vi "LocalizationFGV.vi"(0 "Action":T1, 1 "Dictionary File Path":path, 5 "VI in":refnum<vi>, 7 "Target Language":string, 9 "Input":string, 11 "error in":errorcluster) -> (4 "CSV String":string, 6 "Dictionary":T2, 8 "Languages":string[](array[string]), 10 "Result":string, 14 "Current Language":string, 15 "error out":errorcluster)   [LabVIEW 2020]
uses:
  Dictionary--Cluster.ctl
  Font -- Cluster.ctl
  Phrase Dictionary Entry -- Cluster.ctl
  Localization FGV Action -- Enum.ctl
  VI Info -- Cluster.ctl
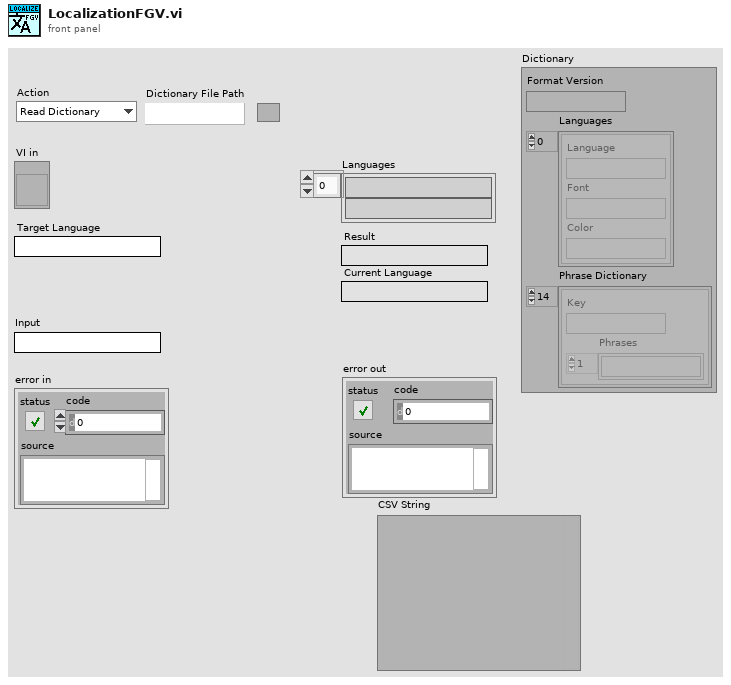
[diagram p1: front panel]
types:
  T1 = typedef "Localization FGV Action -- Enum.ctl" = enum16{"Read Dictionary", "Translate VIs", "Register VI", "Get Languages", "Translate Phrase", "Get Key For Phrase", "Get Phrase For Phrase", "Translate VI", "Unregister"}
  T2 = typedef "Dictionary--Cluster.ctl" = cluster{"Format Version":string, "Languages":T3[], "Phrase Dictionary":T4[]}
  T3 = typedef "Font -- Cluster.ctl" = cluster{"Language":string, "Font":string, "Color":string}
  T4 = typedef "Phrase Dictionary Entry -- Cluster.ctl" = cluster{"Key":string, "Phrases":string[]}
  T5 = typedef "VI Info -- Cluster.ctl" = cluster{"VI Ref":refnum<vi>, "Language":string}
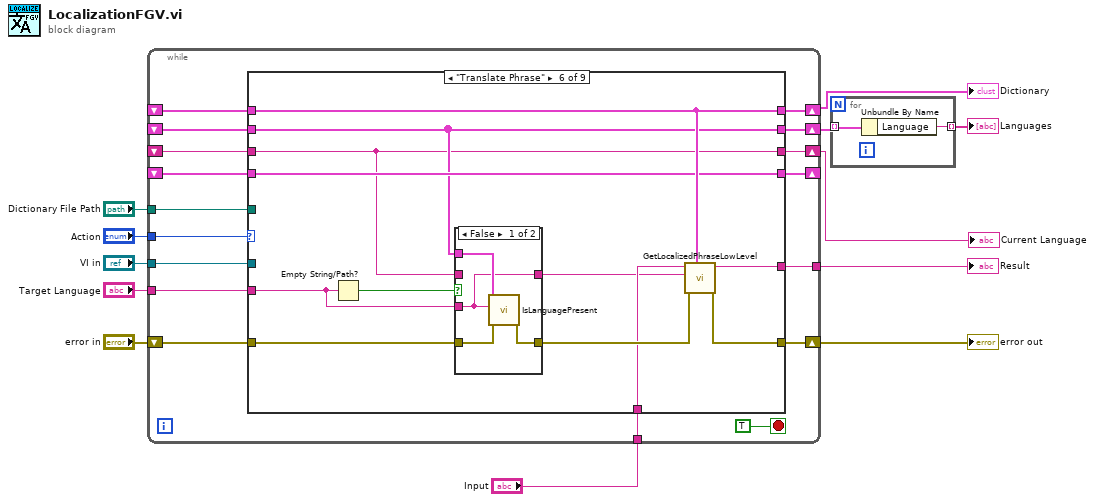
[diagram p0: block diagram]
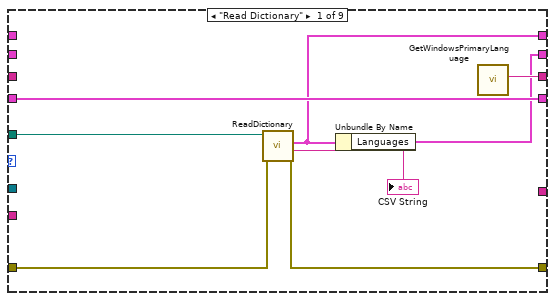
[diagram p2: hidden frame]
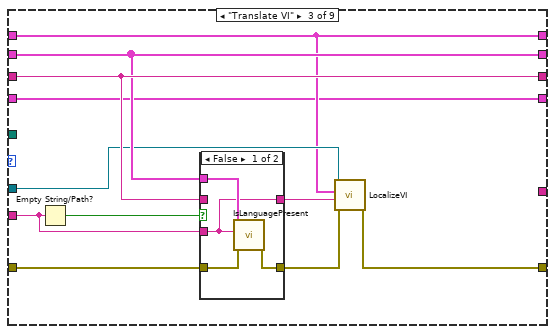
[diagram p4: hidden frame]
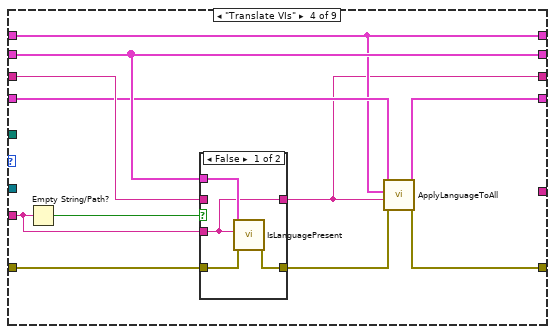
[diagram p6: hidden frame]
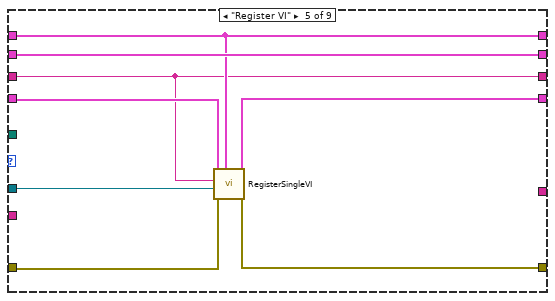
[diagram p8: hidden frame]
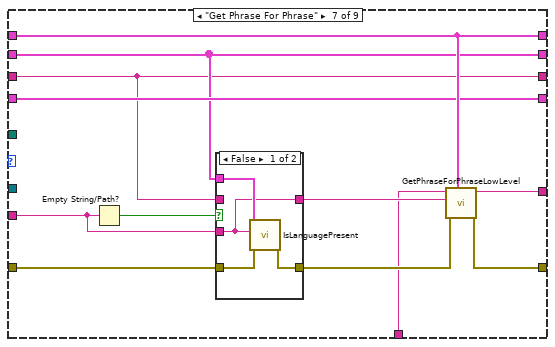
[diagram p10: hidden frame]
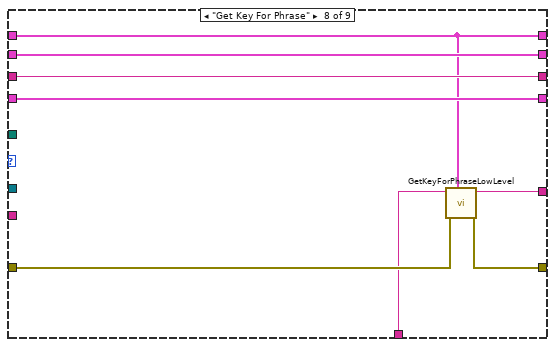
[diagram p12: hidden frame]
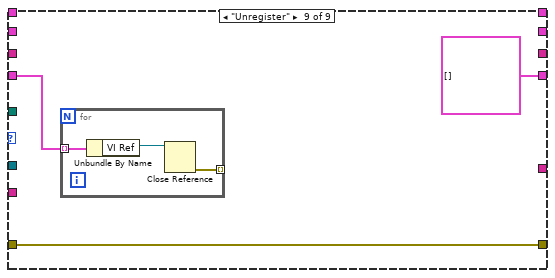
[diagram p13: hidden frame]
diagram:
  n1 = while {
    tunnel: "Action" -> [w28]
    tunnel: "Dictionary File Path" -> [w27]
    shift-right: [w26] -> w4
    shift-left: _ -> [w25]
    shift-right: [w15] -> w11
    shift-left: "error in" -> [w24]
    tunnel: "VI in" -> [w23]
    shift-right: [w22] -> _
    shift-left: _ -> [w21]
    shift-right: [w20] -> w3
    shift-left: _ -> [w19]
    tunnel: "Target Language" -> [w18]
    shift-right: [w17] -> w5
    shift-left: _ -> [w16]
    tunnel: [w14] -> w7
    tunnel: "Input" -> [w13]
    stop <- TRUE stop-if-true
    n2 = case shown="\"Translate Phrase\"" w28 {
      tunnel: w27 -> [w37 _ _ _ _ _ _ _ _]
      tunnel: [w32 w42 w45 w63 w81 w96 w114 w123 _] -> w26
      tunnel: w25 -> [_ w42 w45 w63 w81 w96 w114 w123 _]
      tunnel: w24 -> [w35 w39 w49 w66 w83 w92 w110 w125 w131]
      tunnel: w23 -> [_ _ w46 _ w77 _ _ _ _]
      tunnel: [w34 w40 w43 w64 w79 w94 w112 w128 T5[] [] ("VI Status")] -> w22
      tunnel: w21 -> [w34 w40 w43 w65 w80 w94 w112 w128 w130]
      tunnel: [w31 w41 w50 w67 w84 w90 w108 w127 _] -> w20
      tunnel: w19 -> [_ w41 w50 w67 w84 w90 w108 w127 _]
      tunnel: w18 -> [_ _ w51 w68 _ w89 w106 _ _]
      tunnel: [w33 w38 w52 w60 w78 w88 w105 w126 _] -> w17
      tunnel: w16 -> [_ w38 w52 w69 w78 w88 w105 w126 _]
      tunnel: [w36 w39 w47 w61 w82 w95 w113 w124 w131] -> w15
      tunnel: [_ _ _ _ _ w93 w111 w121 _] -> w14
      tunnel: w13 -> [_ _ _ _ _ w87 w103 w122 _]
      frame "Read Dictionary" {
        n3 = call "ReadDictionary.vi"("error in (no error)"=w35, "Dictionary File Path"=w37) -> ("error out"=w36:errorcluster, "CSV String"=→"CSV String":string, "Dictionary"=w32:T2)  [unwired: 6 in, 1 out]
        n4 = Unbundle By Name(w32) -> ("Languages"=w31:T3[])
        n5 = call "GetWindowsPrimaryLanguage.vi"() -> ("Primary Language"=w33:string)  [unwired: 11 in]
      }
      frame "Get Languages" {
      }
      frame "Translate VI" {
        n6 = Empty String/Path?(string/path=w51) -> (empty?=w53:bool)
        n7 = case shown="False" w53 {
          tunnel: [w55 w58] -> w44
          tunnel: w52 -> [_ w58]
          tunnel: w51 -> [w55 _]
          tunnel: w50 -> [w57 _]
          tunnel: w49 -> [w56 w59]
          tunnel: [w54 w59] -> w48
          frame False {
            n8 = call "IsLanguagePresent.vi"("error in"=w56, "Target Language"=w55, "Languages"=w57) -> ("error out"=w54:errorcluster)  [unwired: 7 in, 1 out]
          }
          frame True {
          }
        }
        n9 = call "LocalizeVI.vi"("error in (no error)"=w48, "Target Language"=w44, "Dictionary"=w45, "VI in"=w46) -> ("error out"=w47:errorcluster)  [unwired: 7 in]
      }
      frame "Translate VIs" {
        n10 = Empty String/Path?(string/path=w68) -> (empty?=w70:bool)
        n11 = case shown="False" w70 {
          tunnel: [w72 w75] -> w60
          tunnel: w69 -> [_ w75]
          tunnel: w68 -> [w72 _]
          tunnel: w67 -> [w74 _]
          tunnel: w66 -> [w73 w76]
          tunnel: [w71 w76] -> w62
          frame False {
            n12 = call "IsLanguagePresent.vi"("error in"=w73, "Target Language"=w72, "Languages"=w74) -> ("error out"=w71:errorcluster)  [unwired: 7 in, 1 out]
          }
          frame True {
          }
        }
        n13 = call "ApplyLanguageToAll.vi"("error in (no error)"=w62, "Target Language"=w60, "Dictionary"=w63, "VI Status"=w65) -> ("error out"=w61:errorcluster, "VI Status"=w64:T5[])  [unwired: 6 in]
      }
      frame "Register VI" {
        n14 = call "RegisterSingleVI.vi"("Dictionary"=w81, "error in (no error)"=w83, "VI in"=w77, "Target Language"=w78, "VI Status"=w80) -> ("Error out"=w82:errorcluster, "VI Status"=w79:T5[])  [unwired: 5 in]
      }
      frame "Translate Phrase" {
        n15 = Empty String/Path?(string/path=w89) -> (empty?=w85:bool)
        n16 = case shown="False" w85 {
          tunnel: [w98 w101] -> w86
          tunnel: w88 -> [_ w101]
          tunnel: w89 -> [w98 _]
          tunnel: w90 -> [w100 _]
          tunnel: w92 -> [w99 w102]
          tunnel: [w97 w102] -> w91
          frame False {
            n17 = call "IsLanguagePresent.vi"("error in"=w99, "Target Language"=w98, "Languages"=w100) -> ("error out"=w97:errorcluster)  [unwired: 7 in, 1 out]
          }
          frame True {
          }
        }
        n18 = call "GetLocalizedPhraseLowLevel.vi"("Dictionary"=w96, "error in (no error)"=w91, "Target Language"=w86, "Key"=w87) -> ("error out"=w95:errorcluster, "Localized Phrase"=w93:string)  [unwired: 5 in, 1 out]
      }
      frame "Get Phrase For Phrase" {
        n19 = Empty String/Path?(string/path=w106) -> (empty?=w107:bool)
        n20 = case shown="False" w107 {
          tunnel: [w116 w119] -> w104
          tunnel: w105 -> [_ w119]
          tunnel: w106 -> [w116 _]
          tunnel: w108 -> [w118 _]
          tunnel: w110 -> [w117 w120]
          tunnel: [w115 w120] -> w109
          frame False {
            n21 = call "IsLanguagePresent.vi"("error in"=w117, "Target Language"=w116, "Languages"=w118) -> ("error out"=w115:errorcluster)  [unwired: 7 in, 1 out]
          }
          frame True {
          }
        }
        n22 = call "GetPhraseForPhraseLowLevel.vi"("Dictionary"=w114, "error in (no error)"=w109, "Target Language"=w104, "Phrase"=w103) -> ("error out"=w113:errorcluster, "Phrase In Target Language"=w111:string)  [unwired: 6 in]
      }
      frame "Get Key For Phrase" {
        n23 = call "GetKeyForPhraseLowLevel.vi"("Dictionary"=w123, "error in (no error)"=w125, "Phrase"=w122) -> ("error out"=w124:errorcluster, "Key"=w121:string)  [unwired: 7 in]
      }
      frame "Unregister" {
        n24 = for {
          tunnel: w130 -> [w134] mode=indexing
          tunnel: [w132] -> _ mode=indexing
          n25 = Unbundle By Name(w134) -> ("VI Ref"=w133:refnum<vi>)
          n26 = Close Reference(reference=w133) -> (error out=w132:errorcluster)  [unwired: 1 in]
        }
      }
    }
  }
  "error out" <- w11
  "Dictionary" <- w4
  "Result" <- w7
  "Current Language" <- w5
  n27 = for {
    tunnel: w3 -> [w136] mode=indexing
    tunnel: [w135] -> w2 mode=indexing
    n28 = Unbundle By Name(w136) -> ("Language"=w135:string)
  }
  "Languages" <- w2
